vi "Odometry Loop.vi"(6 "error in (no error)":errorcluster) -> ()   [LabVIEW 2018]
uses:
  Typedef/Velocity Data.ctl
  Typedef/Odometry.ctl
  Drive/Pure Pursuit/Typedef/Pure Pursuit Telemetry.ctl
  Drive/Pure Pursuit/Typedef/Path Point.ctl
  <vilib>/Rock Robotics/Network Tables/NT Write Number.vi
  <vilib>/Rock Robotics/Network Tables/NT Write Numeric Array.vi
  Drive/Pure Pursuit/Visualization/Current Path.vi
  <vilib>/Platform/TimedLoop/XDataNode/wakeup.ctl
  <vilib>/Platform/TimedLoop/XDataNode/XDNodeRunTimeDep.lvlib
  <vilib>/Platform/TimedLoop/XDataNode/nitl_modes.ctl
  <vilib>/Platform/TimedLoop/XDataNode/timing_clust.ctl
  <vilib>/platform/TimedLoop/XDataNode/XDataNode.xnode
  Drive/Pure Pursuit/Pure Pursuit.lvlib
panel:
  out "Late Iterations":i16
  out "XY Graph":cluster{dbl[], dbl[]}[](graph)=[{array[1000 elements], array[1000 elements]}, {[-2.247939211922799, 9.450601976465425, 8.114176327244312, -3.5843648611439116, -2.247939211922799], [3.8835413402382706, 1.2106900417960451, -4.638580552398066, -1.9657292539558406, 3.8835413402382706]}, {[0.0, 40.0, 60.0, 100.0], [0.0, 20.0, 80.0, 40.0]}, {array[304 elements], array[304 elements]}, {[7.524752475247524, 1.9801980198019802], [-4.118238955689372, -1.1545613507952672]}, {[-5.727080057823512, -5.705598316147173, -5.641285533198998, -5.534538218672029, -5.386014505257412, -5.196630091037495, -4.967552593902651, -4.700194352798713, -4.396203720187724, -4.057454899406876, -3.686036389581695, -3.28423810933444, -2.8545372786743237, -2.3995831461123918, -1.922180655163488, -1.4252731509367513, -0.9119242334342519, -0.38529886943823066, 0.15135612056157366, 0.6947320800959187, 1.241478915683433, 1.7882257512709472, 2.331601710805292, 2.8682567008050963, 3.3948820648011178, 3.9082309823036177, 4.405138486530354, 4.882540977479257, 5.337495110041189, 5.767195940701306, 6.16899422094856, 6.540412730773742, 6.87916155155459, 7.1831521841655785, 7.450510425269517, 7.679587922404362, 7.86897233662428, 8.017496050038897, 8.124243364565864, 8.18855614751404, 8.210037889190378, 8.18855614751404, 8.124243364565865, 8.017496050038897, 7.86897233662428, 7.679587922404362, 7.450510425269517, 7.18315218416558, 6.879161551554592, 6.540412730773744, 6.168994220948562, 5.76719594070131, 5.337495110041191, 4.882540977479256, 4.405138486530356, 3.9082309823036216, 3.3948820648011195, 2.868256700805095, 2.3316017108052938, 1.788225751270952, 1.2414789156834347, 0.6947320800959172, 0.15135612056157544, -0.3852988694382258, -0.9119242334342501, -1.4252731509367527, -1.9221806551634866, -2.3995831461123878, -2.854537278674323, -3.2842381093344417, -3.686036389581693, -4.057454899406872, -4.396203720187724, -4.700194352798713, -4.967552593902649, -5.196630091037493, -5.386014505257412, -5.534538218672031, -5.641285533198998, -5.705598316147173, -5.727080057823512], [-7.13175642584397, -7.6785032614314845, -8.22187922096583, -8.758534210965633, -9.285159574961655, -9.798508492464155, -10.295415996690892, -10.772818487639794, -11.227772620201726, -11.657473450861843, -12.059271731109098, -12.430690240934279, -12.769439061715127, -13.073429694326116, -13.340787935430054, -13.5698654325649, -13.759249846784815, -13.907773560199434, -14.0145208747264, -14.078833657674576, -14.100315399350915, -14.078833657674576, -14.0145208747264, -13.907773560199434, -13.759249846784817, -13.5698654325649, -13.340787935430054, -13.073429694326116, -12.769439061715127, -12.430690240934279, -12.0592717311091, -11.657473450861843, -11.227772620201728, -10.772818487639796, -10.295415996690892, -9.798508492464155, -9.285159574961655, -8.758534210965635, -8.22187922096583, -7.678503261431485, -7.131756425843971, -6.5850095902564565, -6.041633630722112, -5.504978640722308, -4.978353276726287, -4.465004359223786, -3.9680968549970497, -3.4906943640481467, -3.035740231486214, -2.6060394008260976, -2.2042411205788426, -1.8328226107536638, -1.4940737899728127, -1.1900831573618227, -0.922724916257887, -0.6936474191230433, -0.504263004903124, -0.355739291488506, -0.2489919769615394, -0.18467919401336363, -0.16319745233702498, -0.18467919401336363, -0.24899197696153852, -0.355739291488506, -0.5042630049031231, -0.6936474191230424, -0.9227249162578861, -1.1900831573618218, -1.4940737899728118, -1.832822610753662, -2.2042411205788417, -2.6060394008260923, -3.035740231486211, -3.4906943640481467, -3.9680968549970475, -4.465004359223782, -4.978353276726283, -5.5049786407223085, -6.041633630722109, -6.585009590256451, -7.131756425843968]}]
  out "Drivetrain Chart":T1(graph)
  out "Gyro":dbl(graph)
  out "Encoders":T2(graph)
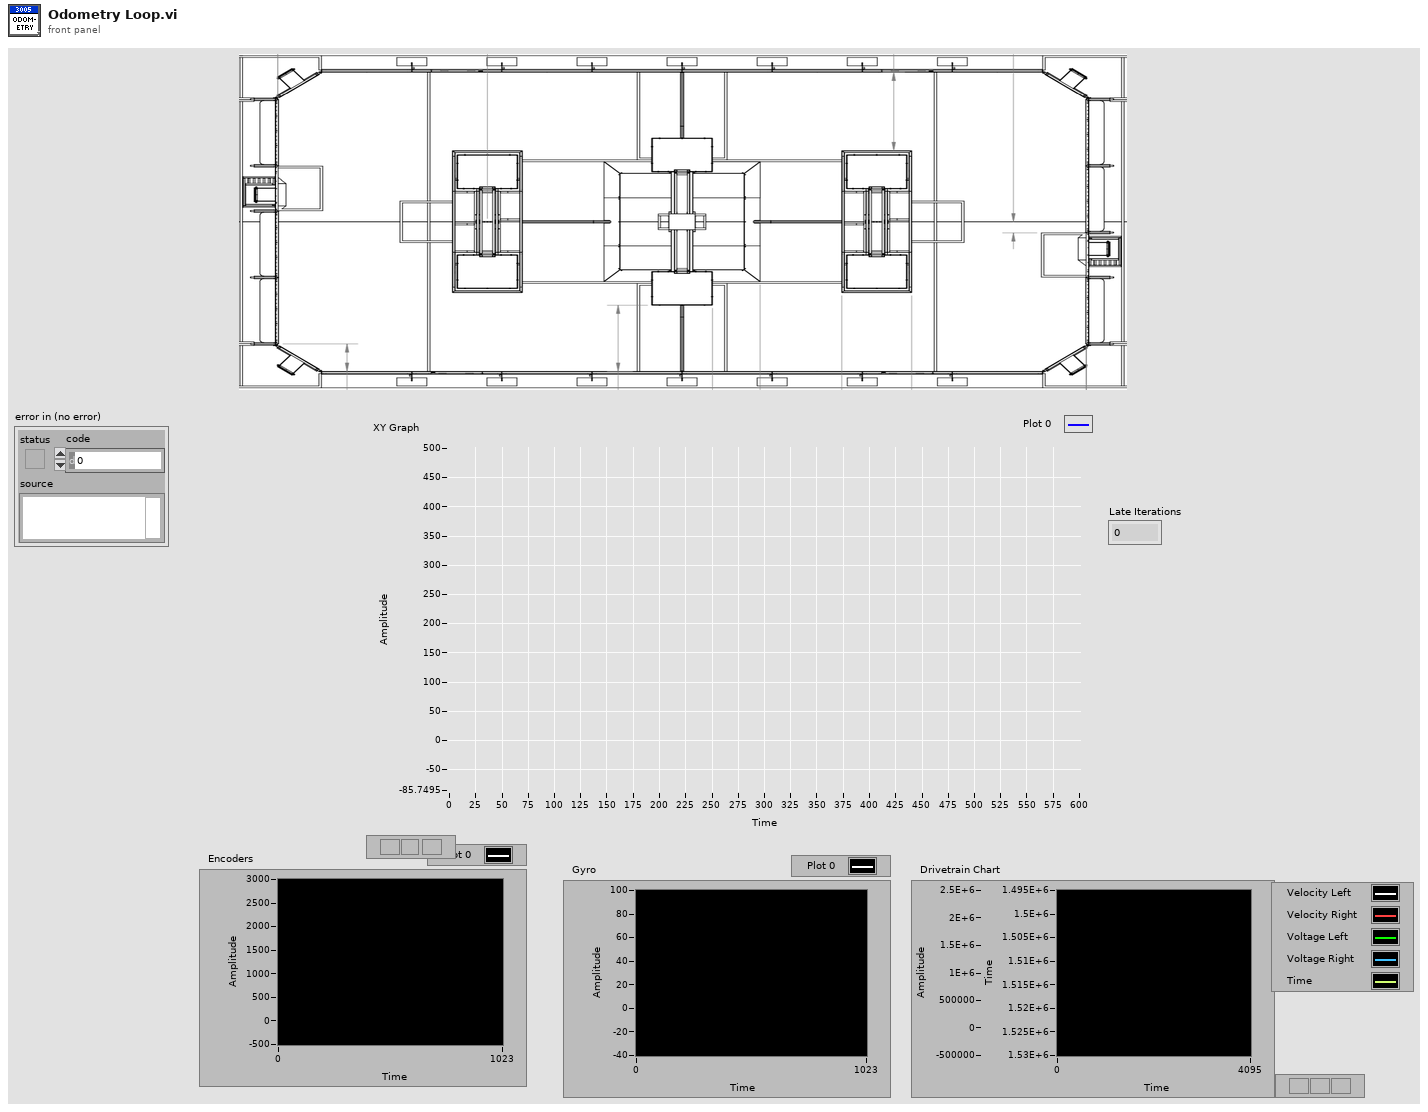
[diagram p1: front panel]
types:
  T1 = cluster{"Left Velocity Raw":sgl, "Right Velocity Raw":sgl, "Voltage":dbl, "Voltage":dbl, "Tick Count(mSec)":u32}
  T2 = cluster{"Left Velocity Raw":sgl, "Right Velocity Raw":sgl}
  T3 = typedef "SPARKMAX6Motor.ctl" = cluster{"FrontLeftMaster":T4, "FrontLeftSlave1":T4, "FrontLeftSlave2":T4, "FrontRightMaster":T4, "FrontRightSlave1":T4, "FrontRightSlave2":T4}
  T4 = typedef "WPI_MotorControlDeviceRef.ctl" = cluster{"DeviceStatus":errorcluster, "Type":T5, "PWM":cluster{"PWM Channel":T6, "DeadBand":T7}, "CAN":cluster{"Device Number":u8, "SetOutput VI Ref":variant, "GetOutput VI Ref":variant, "Enable VI Ref":variant, "Disable VI Ref":variant, "Data":variant}, "Invert":bool, "DIO PWM":cluster{"PWM \"Enable\" Channel":T6, "DIOChannel":T8, "PWM Rate":dbl}}
  T5 = typedef "WPI_MotorControlType.ctl" = enum16{"PWM", "CAN", "DIO PWM"}
  T6 = typedef "FPGA_DIOPWMChannel.ctl" = enum8{"PWM 0", "PWM 1", "PWM 2", "PWM 3", "PWM 4", "PWM 5", "PWM 6", "PWM 7", "PWM 8", "PWM 9", "PWM MXP 0", "PWM MXP 1", "PWM MXP 2", "PWM MXP 3", "PWM MXP 4", "PWM MXP 5", "PWM MXP 6", "PWM MXP 7", "PWM MXP 8", "PWM MXP 9", "Invalid"}
  T7 = typedef "WPI_PWMDeadband.ctl" = cluster{"Name":string, "maxPositivePwm":i32, "minPositivePwm":i32, "centerPwm":i32, "maxNegativePwm":i32, "minNegativePwm":i32, "angularRange":u16}
  T8 = typedef "FPGA_DIOChannel.ctl" = enum8{"DIO 0", "DIO 1", "DIO 2", "DIO 3", "DIO 4", "DIO 5", "DIO 6", "DIO 7", "DIO 8", "DIO 9", "DIO MXP 0", "DIO MXP 1", "DIO MXP 2", "DIO MXP 3", "DIO MXP 4", "DIO MXP 5", "DIO MXP 6", "DIO MXP 7", "DIO MXP 8", "DIO MXP 9", "DIO MXP 10", "DIO MXP 11", "DIO MXP 12", "DIO MXP 13", "DIO MXP 14", "DIO MXP 15", "SPI Port CS1", "SPI Port CS2", "SPI Port CS3", "SPI Port MISO", "SPI Port MOSI", "Invalid"}
  T9 = typedef "WPI_GyroDevRef.ctl" = cluster{"DevStatus":errorcluster, "Analog Channel":T10, "Gain (VoltsPerDegree/Second)":dbl, "Gyro Type":enum16{"Analog", "XRS450"}, "Handle":i32, "SPI Bus":T11, "Device Found":bool, "Sample Rate":dbl, "Calibrate On Open":bool, "Offset":dbl}
  T10 = typedef "FPGA_AIChannel.ctl" = enum8{"AI 0", "AI 1", "AI 2", "AI 3", "AI MXP 0", "AI MXP 1", "AI MXP 2", "AI MXP 3", "Invalid"}
  T11 = typedef "spi_bus.ctl" = enum16{"SPI On-Board, CS0", "SPI On-Board, CS1", "SPI On-Board, CS2", "SPI On-Board, CS3", "SPI MXP", "Invalid"}
  T12 = typedef "Odometry.ctl" = cluster{"x":dbl, "y":dbl, "theta":dbl, "Left Encoder":dbl, "Right Encoder":dbl, "Late Iterations":i16}
  T13 = typedef "XDNodeRunTimeDep.lvlib/timing_clust.ctl" = cluster{"Expected End [f-1]":u64, "Actual End [f-1]":u64, "Finished Late? [f-1]":bool, "Expected End [i-1]":u64, "Actual End [i-1]":u64, "Finished Late? [i-1]":bool, "Expected Start [i]":u64, "Actual Start [i]":u64, "Expected Start [f]":u64, "Actual Start [f]":u64, "Source Name":string, "Structure Name":string, "Period":i64, "Deadline":i64, "Offset":i64, "Start":i64, "Priority":i32, "Timeout":i32, "Mode":T14, "Wakeup Reason":T15, "Error":errorcluster, "Source Type":string, "Secondary Source Type":string, "Global End Time":u64, "Global Start Time":u64, "Frame Duration":u64, "Iteration Duration":u64, "Assigned CPU":i32, "I/O Scan Engine Mode":u32}
  T14 = typedef "XDNodeRunTimeDep.lvlib/nitl_modes.ctl" = enum32{"No Change", "Process missed periods, maintain original phase", "Discard missed periods, maintain original phase", "Process missed periods, ignore original phase", "Discard missed periods, ignore original phase"}
  T15 = typedef "XDNodeRunTimeDep.lvlib/wakeup.ctl" = enum32{"Normal", "Aborted", "Asynchronous wakeup", "Timing source error", "Timed loop error", "Timeout"}
  T16 = typedef "Pure Pursuit.lvlib/Pure Pursuit Telemetry.ctl" = cluster{"Target Point":T17, "Close Point":T17, "Curvature":dbl, "index out":i32}
  T17 = typedef "Pure Pursuit.lvlib/Path Point.ctl" = cluster{"x":dbl, "y":dbl, "heading":dbl, "curvature":dbl, "total distance":dbl, "velocity expected":dbl}
  T18 = typedef "Velocity Data.ctl" = cluster{"Right Velocity Raw":sgl, "Left Velocity Raw":sgl}
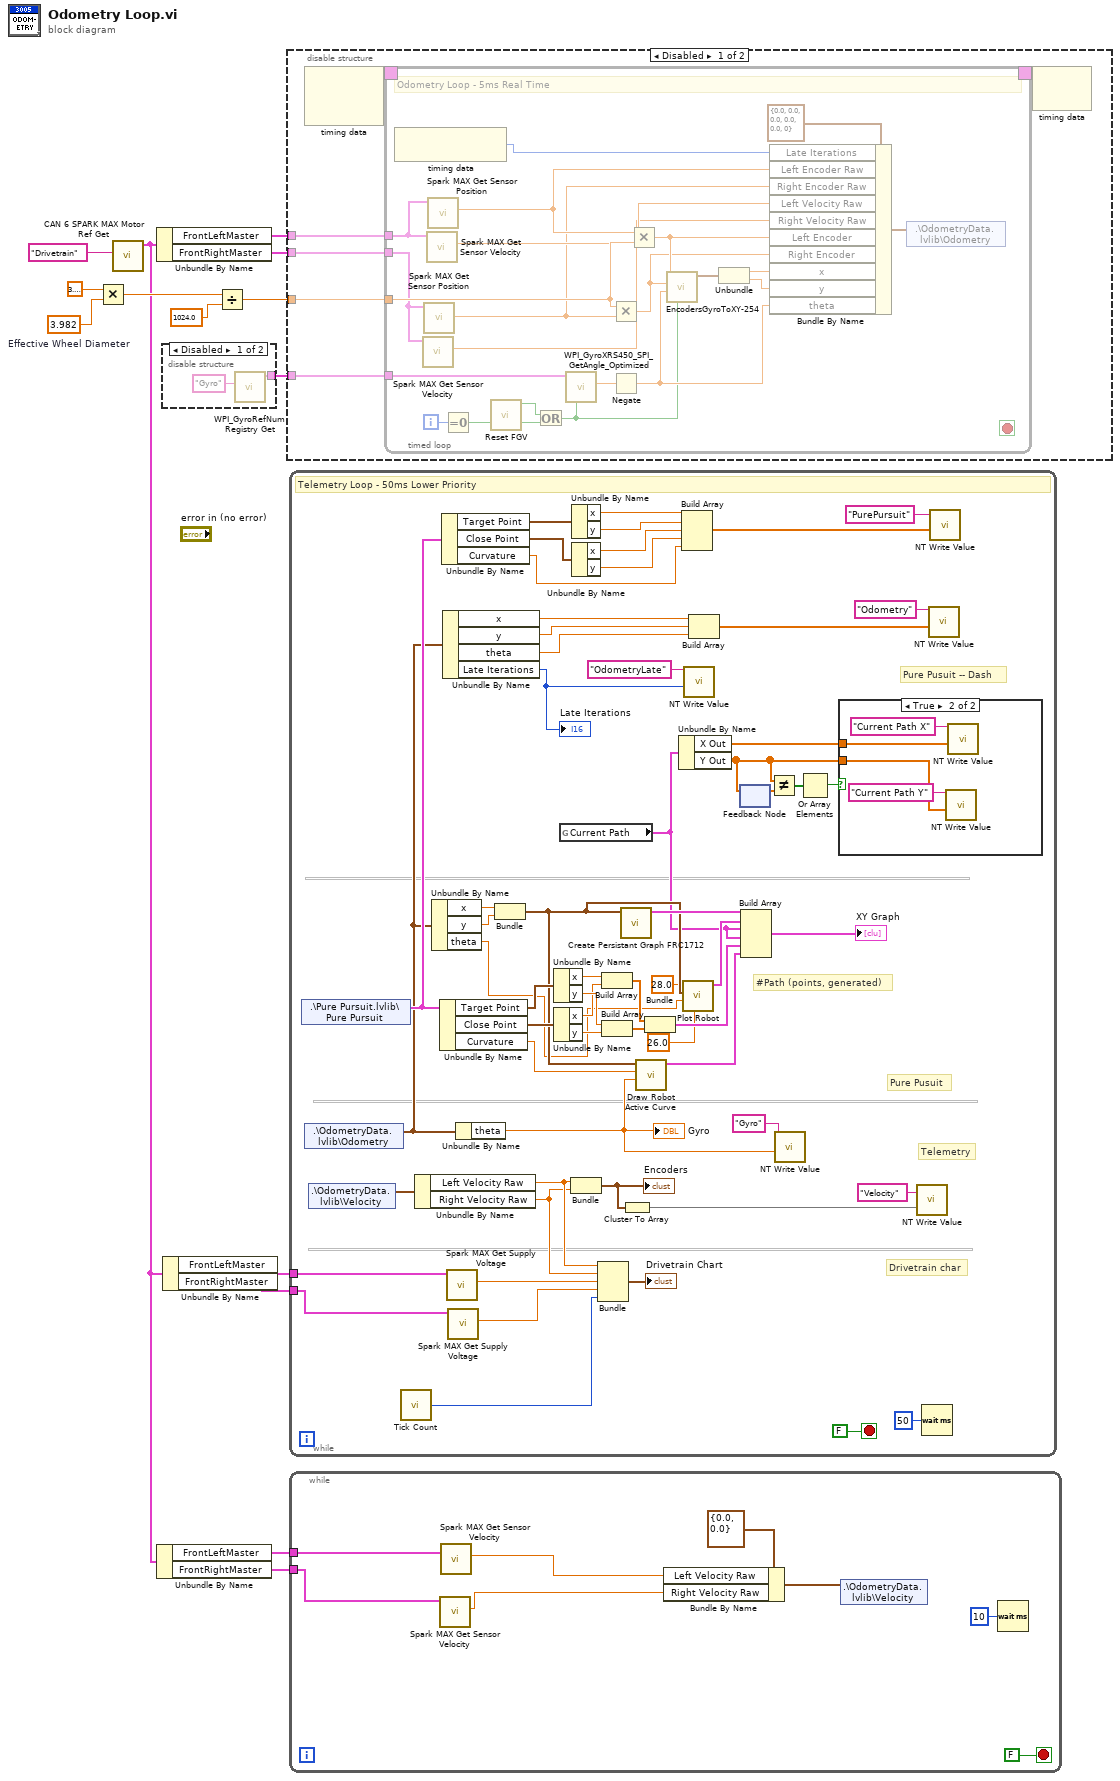
[diagram p0: block diagram]
diagram:
  w8 = 3.982  # Effective Wheel Diameter
  n1 = Multiply(x=3.141592653589793, y=w8) -> (x*y=w6:dbl)
  n2 = call "CAN 6 SPARK MAX Motor Ref Get.vi"("refnum name"="Drivetrain") -> ("TalonSRX6MotorRef out"=w3:T3)  [unwired: 9 in, 1 out]
  n3 = Unbundle By Name(w3) -> ("FrontLeftMaster"=w13:T4, "FrontRightMaster"=w14:T4)
  n4 = Unbundle By Name(w3) -> ("FrontLeftMaster"=w2:T4, "FrontRightMaster"=w1:T4)
  n5 = disable-structure shown="Disabled" {
    disable-tunnel: [w16 _] -> w11
    frame Disabled {
      n6 = call <vilib>:"WPI_GyroRefNum Registry Get.vi"("refnum name"="Gyro") -> ("GyroDevRef"=w16:T9)  [unwired: 9 in, 1 out]
    }
    frame Enabled {
    }
  }
  n7 = Unbundle By Name(w3) -> ("FrontLeftMaster"=w10:T4, "FrontRightMaster"=w9:T4)
  n8 = Divide(x=w6, y=1024.0) -> (x/y=w4:dbl)
  n9 = disable-structure shown="Disabled" {
    disable-tunnel: w14 -> [w20 _]
    disable-tunnel: w13 -> [w19 _]
    disable-tunnel: w11 -> [w18 _]
    disable-tunnel: w4 -> [w17 _]
    frame Disabled {
      n10 = node-c288() -> (w22:T13)  [unwired: 2 in]
      n11 = timed-loop {
        timing: w22 -> [_]
        timing-out: [_] -> w21
        tunnel: w18 -> [w35]
        tunnel: w19 -> [w28]
        tunnel: w20 -> [w25]
        tunnel: w17 -> [w33]
        i -> [w44]
        stop <- _ stop-if-true
        # "Odometry Loop - 5ms Real Time"
        n12 = node-c288() -> (w29:i64)  [unwired: 1 in]
        n13 = call <vilib>:"Spark MAX Get Sensor Velocity.vi"("MotorControlDevRef in"=w25) -> ("Sensor Velocity"=w23:dbl)  [unwired: 7 in, 3 out]
        n14 = call <vilib>:"Spark MAX Get Sensor Position.vi"("MotorControlDevRef in"=w25) -> ("Sensor Position"=w24:dbl)  [unwired: 7 in, 3 out]
        n15 = call <vilib>:"Spark MAX Get Sensor Velocity.vi"("MotorControlDevRef in"=w28) -> ("Sensor Velocity"=w26:dbl)  [unwired: 7 in, 3 out]
        n16 = call <vilib>:"Spark MAX Get Sensor Position.vi"("MotorControlDevRef in"=w28) -> ("Sensor Position"=w27:dbl)  [unwired: 7 in, 3 out]
        n17 = Equal To 0?(x=w44) -> (x = 0?=w31:bool)
        n18 = call "Reset FGV.vi"() -> ("Reset?"=w32:bool)  [unwired: 11 in]
        n19 = Or(x=w32, y=w31) -> (x .or. y?=w30:bool)
        n20 = call "WPI_GyroXRS450_SPI_GetAngle_Optimized.vi"("Reset?"=w30, "GyroDevRef"=w35) -> ("Angle"=w34:dbl)  [unwired: 6 in, 3 out]
        n21 = Multiply(x=w33, y=w24) -> (x*y=w36:dbl)
        n22 = Negate(x=w34) -> (-x=w39:dbl)
        n23 = Multiply(x=w27, y=w33) -> (x*y=w37:dbl)
        n24 = call "EncodersGyroToXY-254.vi"("Reset"=w30, "Angle (degrees)"=w39, "Right Distance"=w36, "Left Distance"=w37) -> ("Location"=w42:cluster{"X":dbl, "Y":dbl})  [unwired: 7 in]
        n25 = Unbundle(w42) -> ("X"=w41:dbl, "Y"=w40:dbl)
        n26 = Bundle By Name(cluster=T12 {"x"=0.0, "y"=0.0, "theta"=0.0, "Left Encoder"=0.0, "Right Encoder"=0.0, "Late Iterations"=0} ("Odometry"), "Late Iterations"=w29, "Left Encoder Raw"=w27, "Right Encoder Raw"=w24, "Left Velocity Raw"=w26, "Right Velocity Raw"=w23, "Left Encoder"=w37, "Right Encoder"=w36, "x"=w41, "y"=w40, "theta"=w39) -> (w38:T12)
        n27 = shared-variable ".\\OdometryData.lvlib\\Odometry"(w38) -> ()  [unwired: 1 in, 1 out]
      }
      n28 = node-c288(w21) -> ()  [unwired: 1 out]
    }
    frame Enabled {
    }
  }
  n29 = while {
    tunnel: w10 -> [w56]
    tunnel: w9 -> [w53]
    stop <- FALSE stop-if-true
    # "Pure Pusuit -- Dash"
    # "Telemetry"
    # "Drivetrain char"
    # "Pure Pusuit"
    # "#Path (points, generated)"
    # "Telemetry Loop - 50ms Lower Priority"
    n30 = shared-variable ".\\Pure Pursuit.lvlib\\Pure Pursuit"() -> (w78:T16)  [unwired: 1 in, 1 out]
    n31 = shared-variable ".\\OdometryData.lvlib\\Odometry"() -> (w69:T12)  [unwired: 1 in, 1 out]
    n32 = shared-variable ".\\OdometryData.lvlib\\Velocity"() -> (w52:T18)  [unwired: 1 in, 1 out]
    n33 = call "Tick Count"() -> ("Tick Count(mSec)"=w84:u32)
    n34 = Unbundle By Name(w52) -> ("Left Velocity Raw"=w51:sgl, "Right Velocity Raw"=w50:sgl)
    n35 = Unbundle By Name(w69) -> ("x"=w104:dbl, "y"=w103:dbl, "theta"=w86:dbl)
    n36 = Unbundle By Name(w78) -> ("Target Point"=w93:T17, "Close Point"=w92:T17, "Curvature"=w91:dbl)
    n37 = Unbundle By Name(w78) -> ("Target Point"=w77:T17, "Close Point"=w76:T17, "Curvature"=w71:dbl)
    n38 = Unbundle By Name(w69) -> ("x"=w68:dbl, "y"=w67:dbl, "theta"=w66:dbl, "Late Iterations"=w57:i16)
    "Late Iterations" <- w57
    n39 = call <vilib>:"Spark MAX Get Supply Voltage.vi"("MotorControlDevRef in"=w56) -> ("Voltage"=w55:dbl)  [unwired: 7 in, 3 out]
    n40 = call <vilib>:"Spark MAX Get Supply Voltage.vi"("MotorControlDevRef in"=w53) -> ("Voltage"=w54:dbl)  [unwired: 7 in, 3 out]
    n41 = Unbundle By Name(w69) -> ("theta"=w89:dbl)
    "Gyro" <- w89
    n42 = Bundle("x"=w104, "y"=w103) -> (w88:cluster{"x":dbl, "y":dbl})  [unwired: 1 in]
    n43 = Unbundle By Name(w93) -> ("x"=w100:dbl, "y"=w99:dbl)
    n44 = Unbundle By Name(w92) -> ("x"=w96:dbl, "y"=w95:dbl)
    n45 = global read "Current Path.vi" "Current Path"() -> (w64:cluster{"X Out":dbl[], "Y Out":dbl[]})
    n46 = Bundle("Left Velocity Raw"=w51, "Right Velocity Raw"=w50) -> (w82:T2)  [unwired: 1 in]
    "Encoders" <- w82
    n47 = Unbundle By Name(w77) -> ("x"=w75:dbl, "y"=w74:dbl)
    n48 = Unbundle By Name(w76) -> ("x"=w73:dbl, "y"=w72:dbl)
    n49 = Bundle("Left Velocity Raw"=w51, "Right Velocity Raw"=w50, "Voltage"=w55, "Voltage"=w54, "Tick Count(mSec)"=w84) -> (→"Drivetrain Chart":T1)  [unwired: 1 in]
    n50 = Build Array(w100, w96) -> (w97:dbl[])
    n51 = Build Array(w99, w95) -> (w98:dbl[])
    n52 = call "Create Persistant Graph FRC1712.vi"("XY"=w88) -> ("Graph Plot"=w107:cluster{dbl[], dbl[]})  [unwired: 10 in]
    n53 = Cluster To Array(cluster=w82) -> (array=w81:sgl[])
    n54 = call "Draw Robot Active Curve.vi"("theta"=w89, "Curvature"=w91, "Cluster"=w88) -> ("circle"=w90:cluster{dbl[], dbl[]})  [unwired: 8 in]
    n55 = Bundle(w97, w98) -> (w94:cluster{dbl[], dbl[]})  [unwired: 1 in]
    n56 = Unbundle By Name(w64) -> ("X Out"=w63:dbl[], "Y Out"=w61:dbl[])
    n57 = Build Array(w75, w74, w73, w72, w71) -> (w70:dbl[])
    n58 = call "Plot Robot.vi"("Length"=26.0, "Angle"=w86, "Location"=w88, "Width"=28.0) -> ("Cluster"=w101:cluster{"X Out":dbl[], "Y Out":dbl[]})  [unwired: 7 in]
    n59 = call-poly <vilib>:"NT Write Value.vi"("Numeric"=w57, "Name"="OdometryLate") -> ()  [unwired: 9 in, 1 out]
    n60 = Build Array(w68, w67, w66) -> (w65:dbl[])
    n61 = feedback-in #1(w61) -> ()
    n62 = feedback #1() -> (w62:dbl[])  [unwired: 1 in]
    n63 = Build Array(w107, w101, w64, w64, w94, w90) -> (→"XY Graph":cluster{"X Out":dbl[], "Y Out":dbl[]}[])
    n64 = Not Equal?(x=w61, y=w62) -> (x != y?=w60:bool[])
    n65 = call-poly <vilib>:"NT Write Value.vi"("Numeric"=w89, "Name"="Gyro") -> ()  [unwired: 9 in, 1 out]
    n66 = Or Array Elements(Boolean array=w60) -> (logical OR=w59:bool)
    n67 = case shown="True" w59 {
      tunnel: w61 -> [_ w111]
      tunnel: w63 -> [_ w110]
      frame False {
      }
      frame True {
        n68 = call-poly <vilib>:"NT Write Value.vi"("Numeric Array"=w111, "Name"="Current Path Y") -> ()  [unwired: 9 in, 1 out]
        n69 = call-poly <vilib>:"NT Write Value.vi"("Numeric Array"=w110, "Name"="Current Path X") -> ()  [unwired: 9 in, 1 out]
      }
    }
    n70 = call-poly <vilib>:"NT Write Value.vi"("Numeric Array"=w81, "Name"="Velocity") -> ()  [unwired: 9 in, 1 out]
    n71 = Wait (ms)(milliseconds to wait=u32 50) -> ()  [unwired: 1 out]
    n72 = call-poly <vilib>:"NT Write Value.vi"("Numeric Array"=w65, "Name"="Odometry") -> ()  [unwired: 9 in, 1 out]
    n73 = call-poly <vilib>:"NT Write Value.vi"("Numeric Array"=w70, "Name"="PurePursuit") -> ()  [unwired: 9 in, 1 out]
  }
  n74 = while {
    tunnel: w2 -> [w119]
    tunnel: w1 -> [w118]
    stop <- FALSE stop-if-true
    n75 = call <vilib>:"Spark MAX Get Sensor Velocity.vi"("MotorControlDevRef in"=w118) -> ("Sensor Velocity"=w117:dbl)  [unwired: 7 in, 3 out]
    n76 = call <vilib>:"Spark MAX Get Sensor Velocity.vi"("MotorControlDevRef in"=w119) -> ("Sensor Velocity"=w116:dbl)  [unwired: 7 in, 3 out]
    n77 = Bundle By Name(cluster=T18 {"Right Velocity Raw"=0.0, "Left Velocity Raw"=0.0} ("Velocity"), "Left Velocity Raw"=w116, "Right Velocity Raw"=w117) -> (w115:T18)
    n78 = shared-variable ".\\OdometryData.lvlib\\Velocity"(w115) -> ()  [unwired: 1 in, 1 out]
    n79 = Wait (ms)(milliseconds to wait=u32 10) -> ()  [unwired: 1 out]
  }
